vi "_Read No Objects.vi"(8 "error in (no error)":errorcluster, 11 "Power Meter in":T1={"Wavelength"=0.0, "AVG"=0, "Range"=0, "Backlight"=0, "Beeper"=0, "Zero"=0, "Local Lockout"=0, "ATTN"=0, "Run/Stop"=0, "Units"=0, "Averaging Time"=0.0, "Averaging"=TRUE, "Most Recent Power"=0.0, "Filter"=0}) -> (0 "error out":errorcluster, 2 "X array":T2, 3 "Power Meter Out":T1={"Wavelength"=0.0, "AVG"=0, "Range"=0, "Backlight"=0, "Beeper"=0, "Zero"=0, "Local Lockout"=0, "ATTN"=0, "Run/Stop"=0, "Units"=0, "Averaging Time"=0.0, "Averaging"=TRUE, "Most Recent Power"=0.0, "Filter"=0})   [LabVIEW 2009]
doc: "(Protected, Dynamic, Pure Virtual/Abstract) Perform a measurement and return one or more channels of data. Outsiders should not call this method, but instead the public \"Read Power.vi\".\n\nThis vi compares the current point to the previous and returns 0 if current if more than twice as much as previous. It also creates a warning, error value of 1."
uses:
  Utility Classes/Readable/X array.ctl
  Utility Classes/Readable/X.ctl
  Global/GPIB Numbers.vi
  Newport 1830-C/Newport 1830-C.lvlib
  Utility Classes/Readable/Readable.lvclass
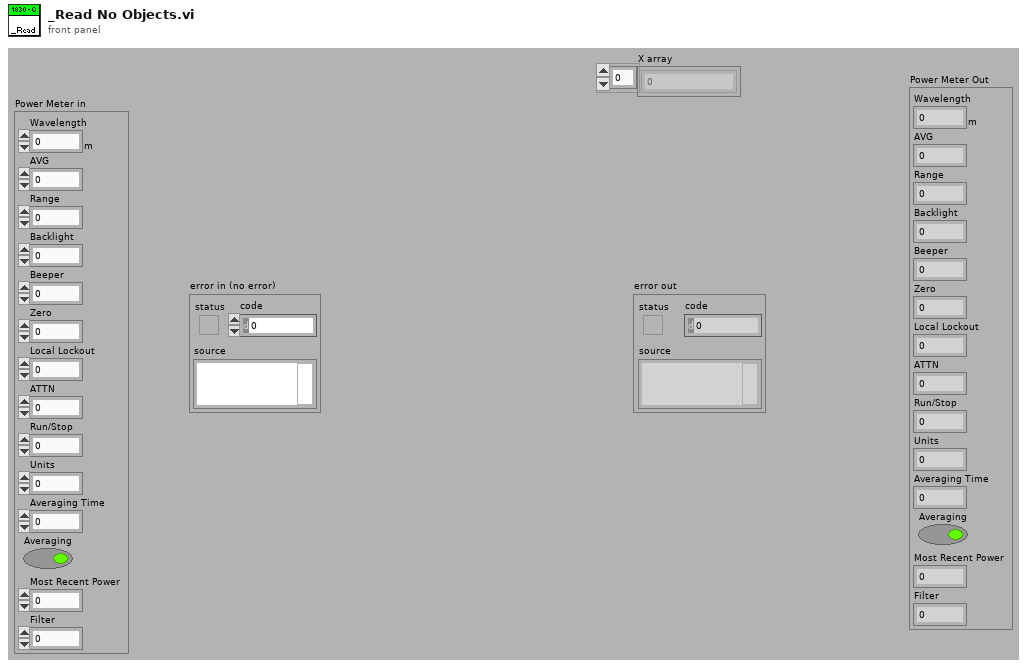
[diagram p1: front panel]
types:
  T1 = cluster{"Wavelength":dbl[unit], "AVG":i32, "Range":i32, "Backlight":i32, "Beeper":i32, "Zero":i32, "Local Lockout":i32, "ATTN":i32, "Run/Stop":i32, "Units":i32, "Averaging Time":dbl, "Averaging":bool, "Most Recent Power":dbl, "Filter":i32}
  T2 = typedef "Readable.lvclass/X array.ctl" = T3[]
  T3 = typedef "Readable.lvclass/X.ctl" = dbl
  T4 = typedef "GPIB Type Def.ctl" = cluster{"Name":string, "bus":dbl, "GPIB":dbl, "GPIB as string":string, "byte":i32, "VISA Resource Name":refnum<visa-resource-name>}
  T5 = typedef "Filters.ctl" = u16
  T6 = cluster{"Wavelength":dbl[unit], "AVG":u16, "Range":u16, "Backlight":u16, "Beeper":u16, "Zero":u16, "Local Lockout":u16, "ATTN":u16, "Run/Stop":u16, "Units":u16, "Averaging Time":dbl, "Averaging":bool, "Most Recent Power":dbl, "Filter":T5}
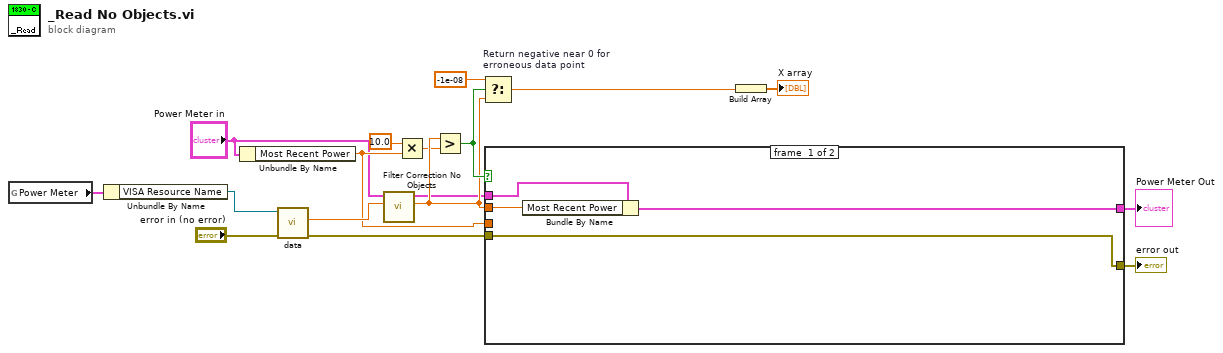
[diagram p0: block diagram]
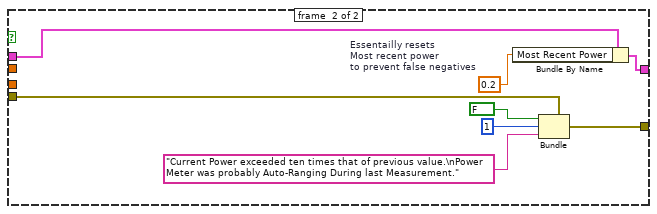
[diagram p2: hidden frame]
diagram:
  n1 = global read "GPIB Numbers.vi" "Power Meter"() -> (w7:T4)
  n2 = Unbundle By Name(w7) -> ("VISA Resource Name"=w6:refnum<visa-resource-name>)
  n3 = Unbundle By Name("Power Meter in") -> ("Most Recent Power"=w8:dbl)
  n4 = call "data.vi"("error in (no error)"="error in (no error)", "VISA resource name"=w6) -> ("error out"=w3:errorcluster, "Power"=w12:dbl)  [unwired: 7 in, 1 out]
  n5 = call "Filter Correction No Objects.vi"("Read Power"=w12, "Cluster In"="Power Meter in") -> ("Corrected Power"=w11:dbl, "Cluster Out"=w2:T6)  [unwired: 8 in]
  n6 = Multiply(x=10.0, y=w8) -> (x*y=w9:dbl)
  n7 = Greater?(x=w11, y=w9) -> (0:w15:bool)
  n8 = Select "Return negative near 0 for\nerroneous data point"(t=-1e-08, s=w15, f=w11) -> (s? t:f=w13:dbl)
  n9 = case shown="True" w15 {
    tunnel: w3 -> [w21 w29]
    tunnel: [w21 w25] -> w14
    tunnel: w2 -> [w20 w24]
    tunnel: w11 -> [w18 _]
    tunnel: [w19 w23] -> w1
    tunnel: w8 -> [_ _]
    frame #0 {
      n10 = Bundle By Name(cluster=w20, "Most Recent Power"=w18) -> (w19:T6)
    }
    frame #1 {
      w22 = 0.2  # Essentailly resets Most recent power to prevent false negatives
      n11 = Bundle By Name(cluster=w24, "Most Recent Power"=w22) -> (w23:T6)
      n12 = Bundle(cluster=w29, "status"=FALSE, "code"=1, "source"="Current Power exceeded ten times that of previous value.\nPower Meter was probably Auto-Ranging During last Measurement.") -> (w25:errorcluster)
    }
  }
  "error out" <- w14
  "Power Meter Out" <- w1
  n13 = Build Array(w13) -> (→"X array":dbl[])
